vi "E2 Data Logger.vi"(7 "refnum in":refnum<file>) -> (3 "refnum out":refnum<file>)   [LabVIEW 2014]
uses:
  <vilib>/Rock Robotics/WPI/DriverStation/WPI_DriverStationRobotMode2.ctl
  Robot Global Data.vi
  GlobalVariable.vi
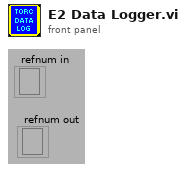
[diagram p1: front panel]
types:
  T1 = typedef "WPI_DriverStationRobotMode2.ctl" = enum16{"Autonomous Disabled", "Autonomous Enabled", "Teleop Disabled", "Teleop Enabled", "Disconnected", "Finish", "Test Disabled", "Test Enabled", "Emergency Stopped"}
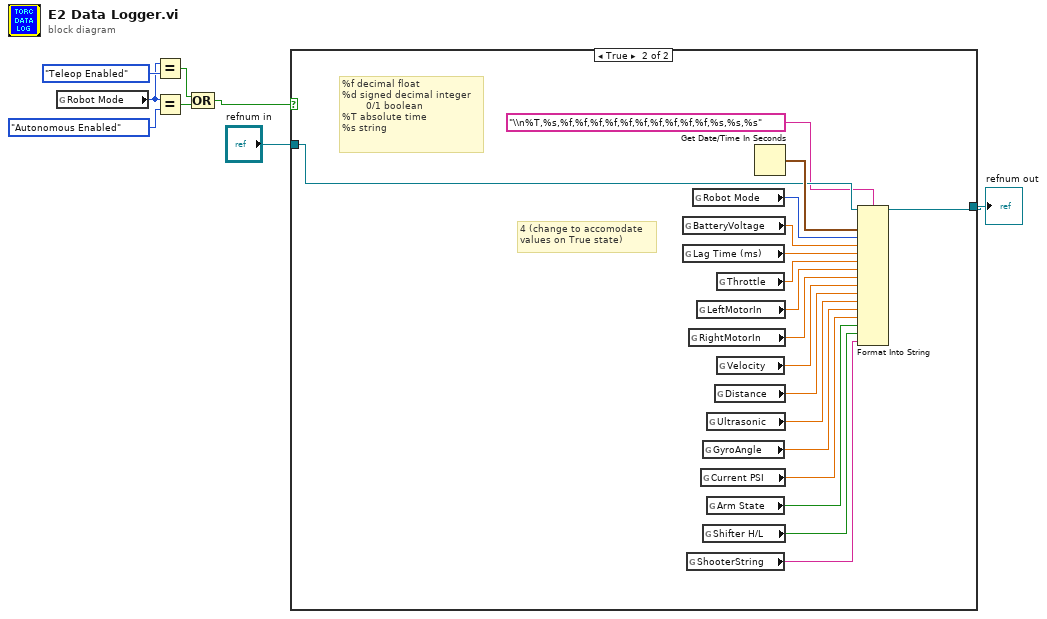
[diagram p0: block diagram]
diagram:
  n1 = global read "Robot Global Data.vi" "Robot Mode"() -> (w1:T1)
  n2 = Equal?(x=w1, y=WPI_DriverStationRobotMode2."Teleop Enabled") -> (x = y?=w4:bool)
  n3 = Equal?(x=w1, y=WPI_DriverStationRobotMode2."Autonomous Enabled") -> (x = y?=w3:bool)
  n4 = Compound Arithmetic op=OR(w4, w3) -> (w2:bool)
  n5 = case shown="True" w2 {
    tunnel: [w9 w27] -> w8
    tunnel: "refnum in" -> [w9 w25]
    frame False {
    }
    frame True {
      # "%f decimal float\n%d signed decimal integer\n        0/1 boolean\n%T absolute time\n%s string"
      # "4 (change to accomodate\nvalues on True state)"
      n6 = global read "GlobalVariable.vi" "BatteryVoltage"() -> (w23:dbl)
      n7 = global read "GlobalVariable.vi" "Lag Time (ms)"() -> (w22:dbl)
      n8 = global read "GlobalVariable.vi" "ShooterString"() -> (w11:string)
      n9 = global read "GlobalVariable.vi" "RightMotorIn"() -> (w19:dbl)
      n10 = global read "Robot Global Data.vi" "Robot Mode"() -> (w24:T1)
      n11 = global read "GlobalVariable.vi" "LeftMotorIn"() -> (w20:dbl)
      n12 = global read "GlobalVariable.vi" "Current PSI"() -> (w14:dbl)
      n13 = global read "GlobalVariable.vi" "GyroAngle"() -> (w15:dbl)
      n14 = global read "GlobalVariable.vi" "Shifter H/L"() -> (w12:bool)
      n15 = global read "GlobalVariable.vi" "Ultrasonic"() -> (w16:dbl)
      n16 = global read "GlobalVariable.vi" "Arm State"() -> (w13:bool)
      n17 = global read "GlobalVariable.vi" "Distance"() -> (w17:dbl)
      n18 = global read "GlobalVariable.vi" "Throttle"() -> (w21:dbl)
      n19 = global read "GlobalVariable.vi" "Velocity"() -> (w18:dbl)
      n20 = Get Date/Time In Seconds() -> (seconds since 1Jan1904=w26:timestamp)
      n21 = Format Into String(format string="\\n%T,%s,%f,%f,%f,%f,%f,%f,%f,%f,%f,%f,%s,%s,%s", initial string=w25, w26, w24, w23, w22, w21, w20, w19, w18, w17, w16, w15, w14, w13, w12, w11) -> (resulting string=w27:refnum<file>)  [unwired: 1 in, 1 out]
    }
  }
  "refnum out" <- w8
